vi "Data To API String Arguments.vi"(7 "reference cluster data":variant, 9 "error in (no error)":errorcluster, 10 "No Tag Mode(F)":bool, 11 "data":variant) -> (1 "error out":errorcluster, 3 "String":string)   [LabVIEW 2017, in "API String Arguments Support.lvlib"]
uses:
  API String Arguments Support.lvlib
  <userlib>/_NEVSTOP/Communicable State Machine(CSM)/AdvanceAPI/CSM - Keywords.vi
  <vilib>/Utility/Data Type/NI_Data Type.lvlib
  <userlib>/_NEVSTOP/Communicable State Machine(CSM)/Communicable State Machine.lvlib
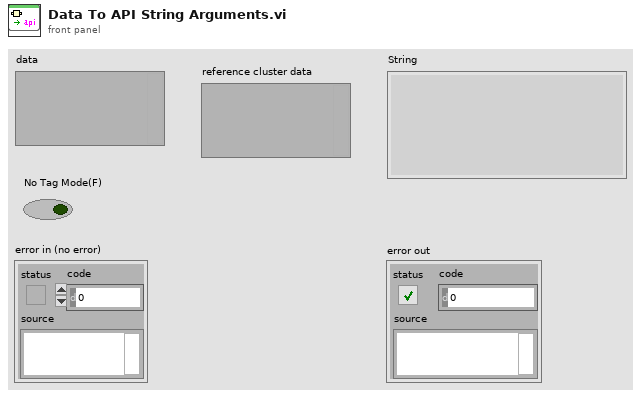
[diagram p1: front panel]
types:
  T1 = typedef "NI_Data Type.lvlib/Data Type.ctl" = enum8{"Invalid Type", "Void", "I8", "I16", "I32", "I64", "U8", "U16", "U32", "U64", "Single Float", "Double Float", "Extended Float", "Single Complex", "Double Complex", "Extended Complex", "Enum U8", "Enum U16", "Enum U32", "Enum U64", "Single Float With Unit", "Double Float With Unit", "Extended Float With Unit", "Single Complex with Unit", "Double Complex with Unit", "Extended Complex with Unit", "Boolean", "String", "Path", "Picture", "Tag", "Array", "Cluster", "Variant", "LV Variant", "Waveform", "Timestamp", "Digital Waveform", "Digital Data", "ExpressData", "Refnum", "External Data", "VI", "Poly VI", "LabVIEW Class Instance", "Fixed Point"}
  T2 = typedef "NI_Data Type.lvlib/Refnum Type.ctl" = enum16{"NotARefnum", "UnknownRefnum", "Generic", "Datalog", "ByteStream", "Device", "Occurence", "TCPNetConnection", "Auto", "Menu", "Imaq", "Hardware", "DataSocket", "Visa", "IVI", "UDPNetConnection", "Notifier", "Queue", "Irda", "EventReg", "DotNet", "UserEvent", "Callback", "UNUSED_EMPTY_POSITION", "BlueToothNetConnection", "LVObjApp", "LVObjVI", "LVObjUnknown", "GenericClass", "UserDefinedRefnumTag", "DataValue", "RT FIFO", "TDMS File"}
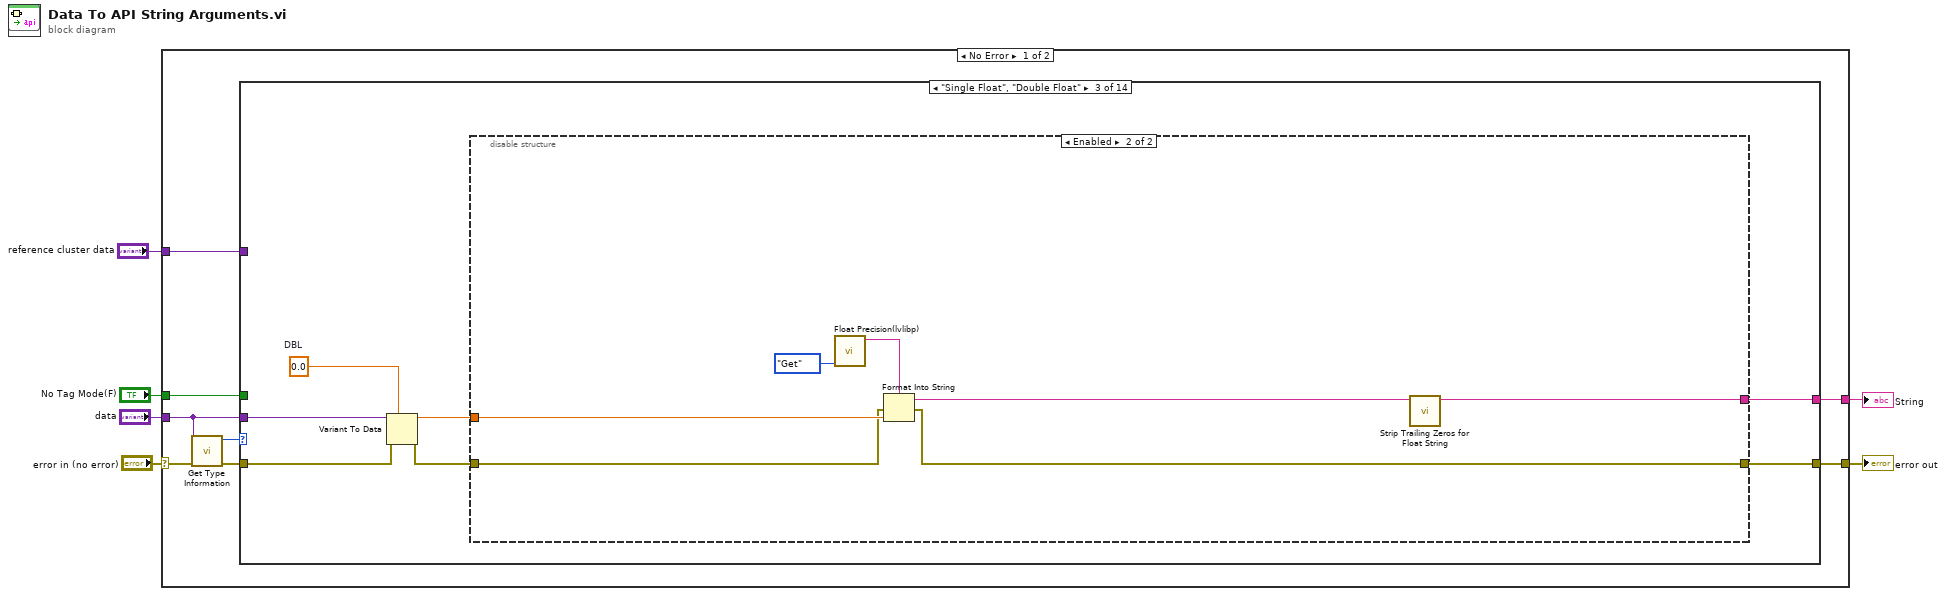
[diagram p0: block diagram]
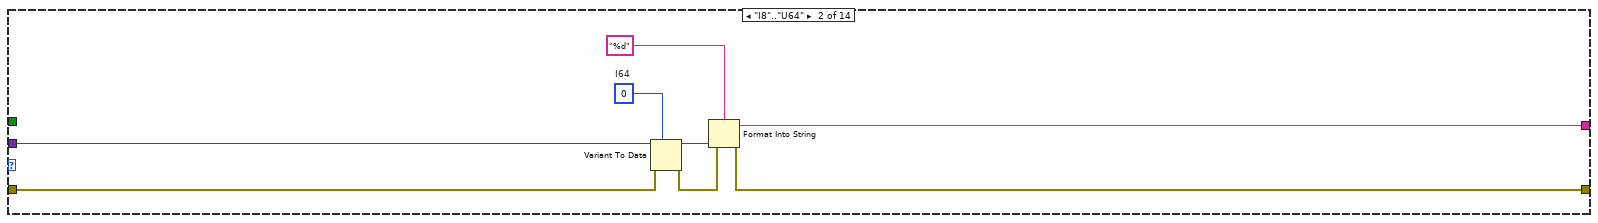
[diagram p3: hidden frame]
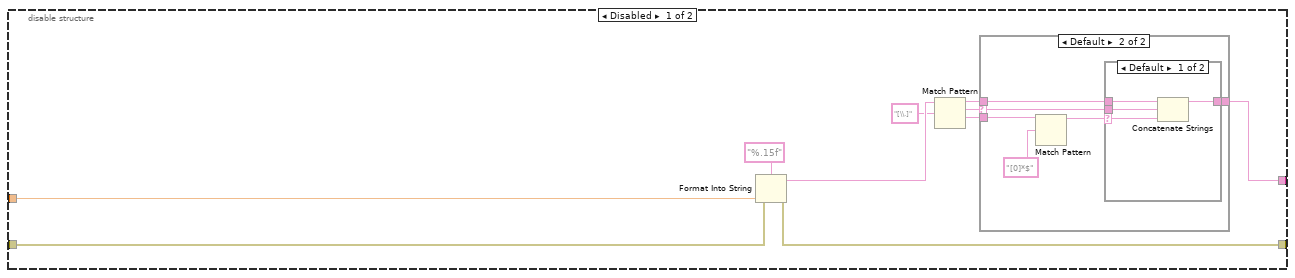
[diagram p4: hidden frame]
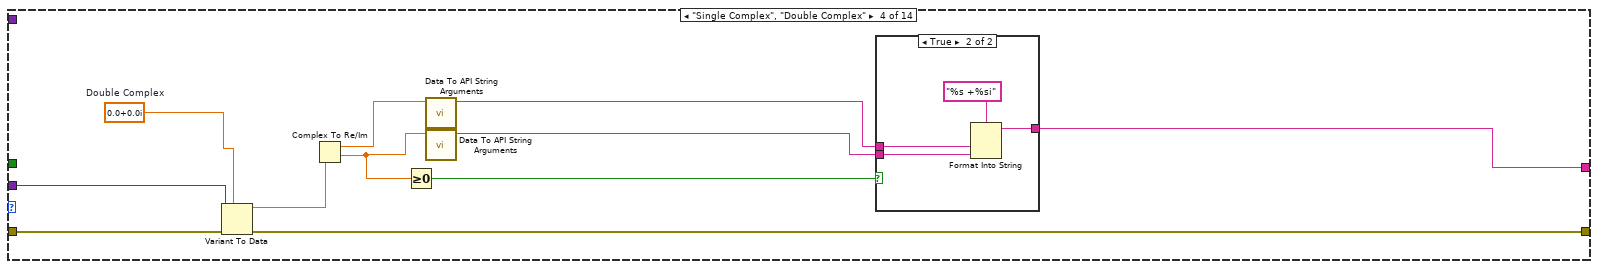
[diagram p7: hidden frame]
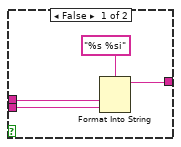
[diagram p8: hidden frame]
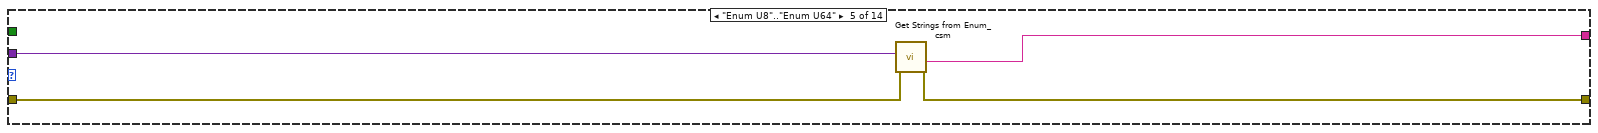
[diagram p9: hidden frame]
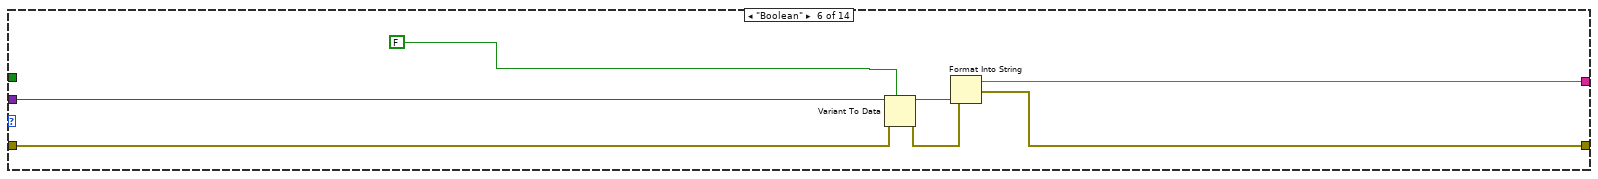
[diagram p10: hidden frame]
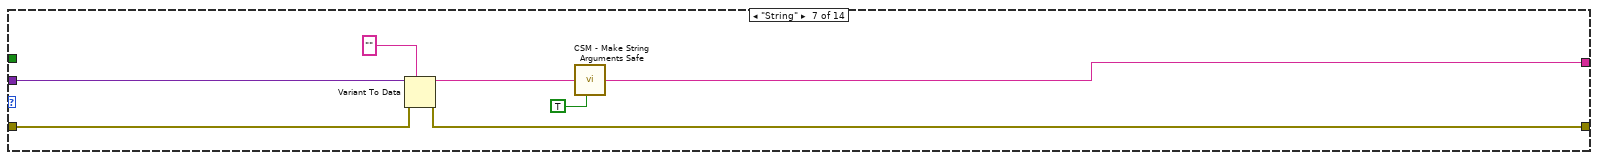
[diagram p11: hidden frame]
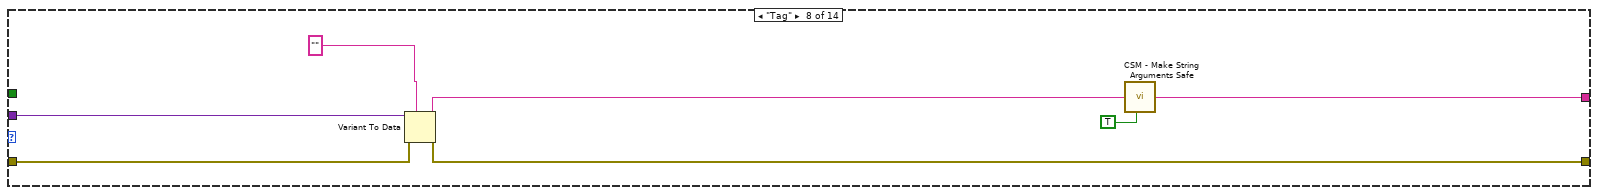
[diagram p12: hidden frame]
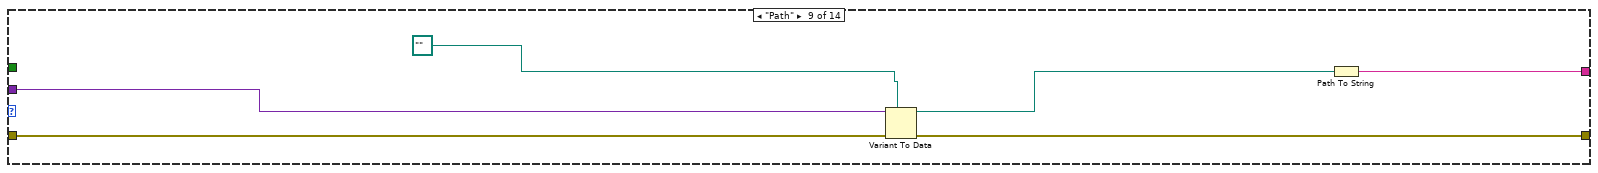
[diagram p13: hidden frame]
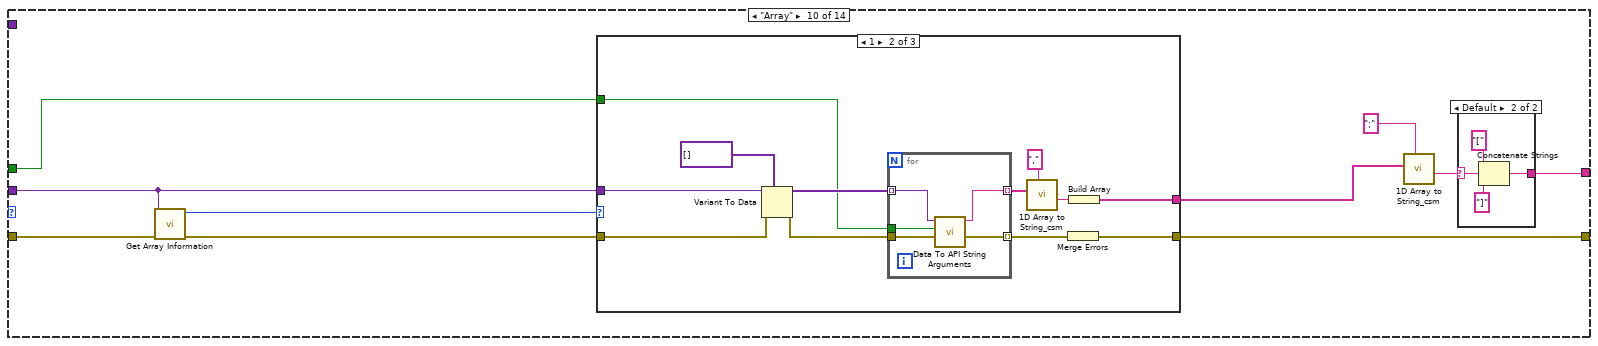
[diagram p14: hidden frame]
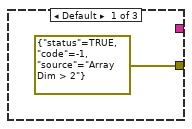
[diagram p15: hidden frame]
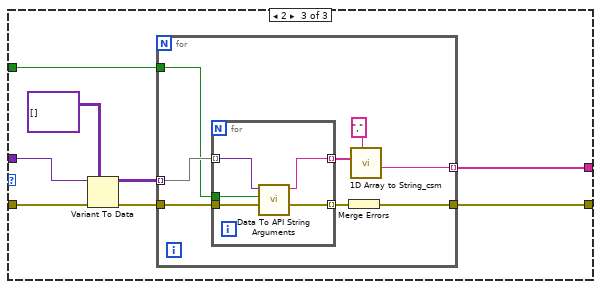
[diagram p16: hidden frame]
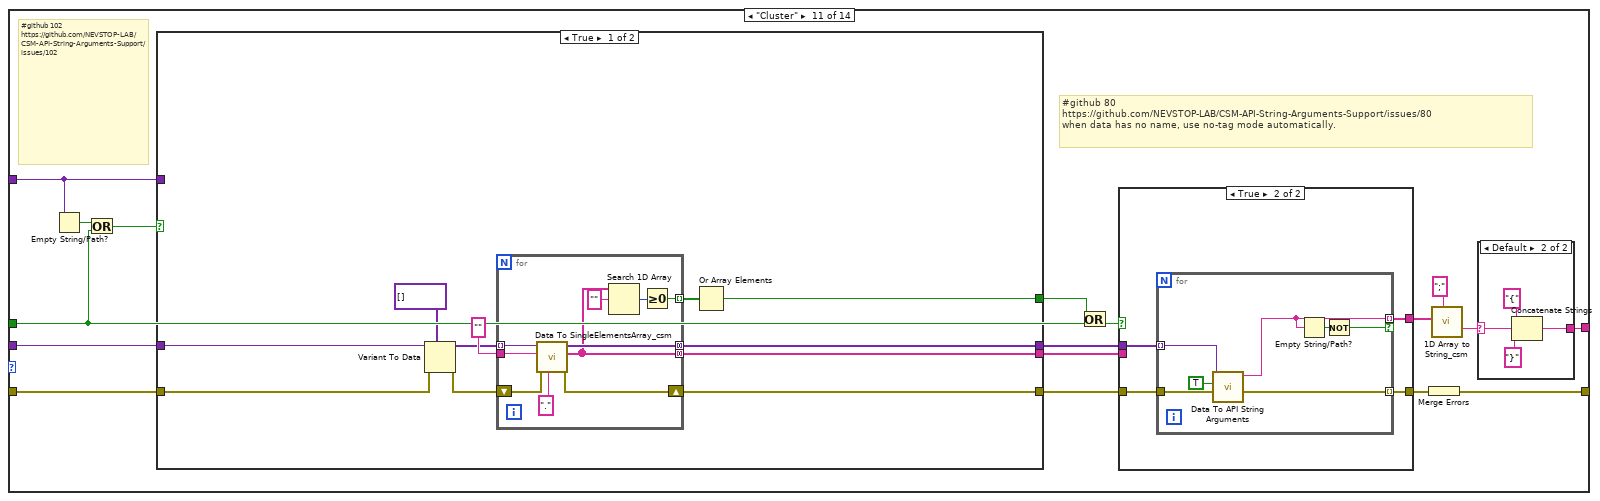
[diagram p18: hidden frame]
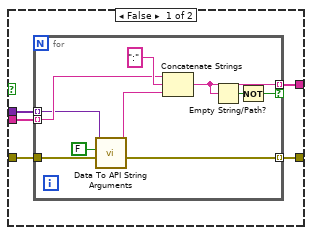
[diagram p19: hidden frame]
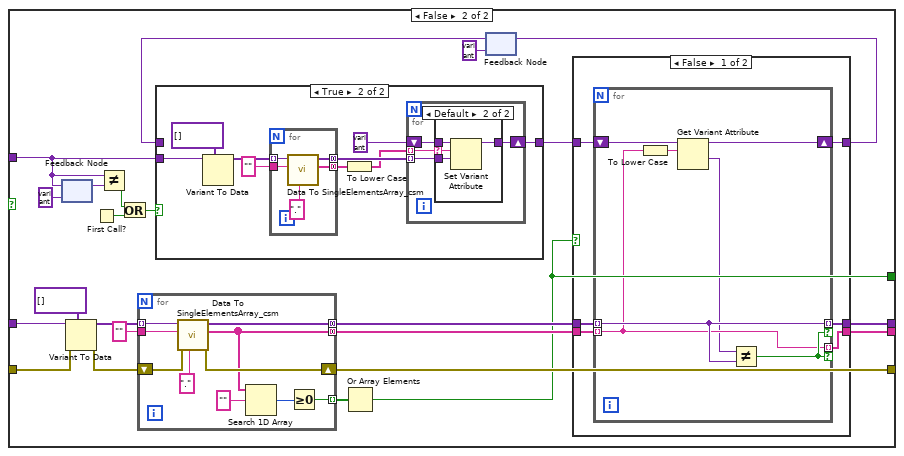
[diagram p20: hidden frame]
diagram:
  n1 = case shown="No Error" "error in (no error)" {
    selector: "error in (no error)" -> [w9 w325]
    tunnel: [w13 _] -> w6
    tunnel: "data" -> [w12 _]
    tunnel: [w10 w325] -> w4
    tunnel: "reference cluster data" -> [w8 _]
    tunnel: "No Tag Mode(F)" -> [w7 _]
    frame No Error {
      n2 = call <vilib>:"Get Type Information.vi"("error in (no error)"=w9, "Variant"=w12) -> ("error out"=w11:errorcluster, "Type"=w14:T1)  [unwired: 5 in, 3 out]
      n3 = case shown="\"Single Float\", \"Double Float\"" w14 {
        tunnel: [_ w19 w24 w65 w81 w87 w91 w98 w104 w119 w179 w304 w310 w319] -> w13
        tunnel: w12 -> [_ w23 w30 w68 w82 w89 w96 w103 w109 w117 w174 w305 w308 w324]
        tunnel: w11 -> [w15 w18 w28 w70 w80 w86 w94 w101 w107 w118 w173 w306 w311 w322]
        tunnel: [w15 w16 w26 w69 w79 w84 w93 w100 w106 w115 w177 w306 w309 w321] -> w10
        tunnel: w8 -> [_ _ _ _ _ _ _ _ _ _ w169 _ _ _]
        tunnel: w7 -> [_ _ _ _ _ _ _ _ _ w110 w163 _ _ _]
        frame "Invalid Type", "Void" {
        }
        frame "I8".."U64" {
          w22 = i64 0  # I64
          n4 = Variant To Data(error in=w18, type=w22, Variant=w23) -> (data=w21:i64, error out=w17:errorcluster)
          n5 = Format Into String(format string="%d", error in=w17, w21) -> (resulting string=w19:string, error out=w16:errorcluster)  [unwired: 1 in]
        }
        frame "Single Float", "Double Float" {
          w25 = 0.0  # DBL
          n6 = Variant To Data(error in=w28, type=w25, Variant=w30) -> (data=w29:dbl, error out=w27:errorcluster)
          n7 = disable-structure shown="Enabled" {
            disable-tunnel: w29 -> [w40 w59]
            disable-tunnel: w27 -> [w38 w58]
            disable-tunnel: [w37 w57] -> w26
            disable-tunnel: [w31 w55] -> w24
            frame Disabled {
              n8 = Format Into String(format string="%.15f", error in=w38, w40) -> (resulting string=w36:string, error out=w37:errorcluster)  [unwired: 1 in]
              n9 = Match Pattern(string=w36, regular expression="[\\.]") -> (before substring=w33:string, match substring=w32:string, after substring=w34:string)  [unwired: 1 in, 1 out]
              n10 = case shown="Default" w32 {
                selector: w32 -> [_ w44]
                tunnel: w34 -> [_ w47]
                tunnel: w33 -> [w41 w45]
                tunnel: [w41 w42] -> w31
                frame "" {
                }
                frame Default {
                  n11 = Match Pattern(string=w47, regular expression="[0]*$") -> (before substring=w43:string)  [unwired: 1 in, 3 out]
                  n12 = case shown="Default" w43 {
                    selector: w43 -> [w49 _]
                    tunnel: w45 -> [w51 w52]
                    tunnel: w44 -> [w50 _]
                    tunnel: [w48 w52] -> w42
                    frame Default {
                      n13 = Concatenate Strings(w51, w50, w49) -> (w48:string)
                    }
                    frame "" {
                    }
                  }
                }
              }
            }
            frame Enabled {
              n14 = call "Float Precision(lvlibp).vi"("Enum"=enum16{"Set", "Get"}."Get") -> ("Format String"=w53:string)  [unwired: 10 in]
              n15 = Format Into String(format string=w53, error in=w58, w59) -> (resulting string=w56:string, error out=w57:errorcluster)  [unwired: 1 in]
              n16 = call "Strip Trailing Zeros for Float String.vi"("Float String"=w56) -> ("Float String with Same Value"=w55:string)  [unwired: 10 in]
            }
          }
        }
        frame "Single Complex", "Double Complex" {
          w67 = cdb 0.0+0.0i  # Double Complex
          n17 = Variant To Data(error in=w70, type=w67, Variant=w68) -> (data=w66:cdb, error out=w69:errorcluster)
          n18 = Complex To Re/Im(x + iy=w66) -> (x=w63:dbl, y=w62:dbl)
          n19 = Greater Or Equal To 0?(x=w62) -> (x >= 0?=w64:bool)
          n20 = call "Data To API String Arguments.vi"("data"=w63) -> ("String"=w61:string)  [unwired: 9 in, 1 out]
          n21 = call "Data To API String Arguments.vi"("data"=w62) -> ("String"=w60:string)  [unwired: 9 in, 1 out]
          n22 = case shown="True" w64 {
            tunnel: w61 -> [w72 w77]
            tunnel: w60 -> [w71 w76]
            tunnel: [w73 w75] -> w65
            frame False {
              n23 = Format Into String(format string="%s %si", w72, w71) -> (resulting string=w73:string)  [unwired: 2 in, 1 out]
            }
            frame True {
              n24 = Format Into String(format string="%s +%si", w77, w76) -> (resulting string=w75:string)  [unwired: 2 in, 1 out]
            }
          }
        }
        frame "Enum U8".."Enum U64" {
          n25 = call <userlib>:"Get Strings from Enum_csm.vi"("error in (no error)"=w80, "Enum"=w82) -> ("error out"=w79:errorcluster, "String Value"=w81:string)  [unwired: 6 in, 2 out]
        }
        frame "Boolean" {
          n26 = Variant To Data(error in=w86, type=FALSE, Variant=w89) -> (data=w88:bool, error out=w85:errorcluster)
          n27 = Format Into String(error in=w85, w88) -> (resulting string=w87:string, error out=w84:errorcluster)  [unwired: 2 in]
        }
        frame "String" {
          n28 = Variant To Data(error in=w94, type="", Variant=w96) -> (data=w95:string, error out=w93:errorcluster)
          n29 = call <userlib>:"CSM - Make String Arguments Safe.vi"("Argument String"=w95, "Ignore Argument Type(F)"=TRUE) -> ("Safe Argument String"=w91:string)  [unwired: 7 in]
        }
        frame "Tag" {
          n30 = Variant To Data(error in=w101, type="", Variant=w103) -> (data=w102:string, error out=w100:errorcluster)
          n31 = call <userlib>:"CSM - Make String Arguments Safe.vi"("Argument String"=w102, "Ignore Argument Type(F)"=TRUE) -> ("Safe Argument String"=w98:string)  [unwired: 7 in]
        }
        frame "Path" {
          n32 = Variant To Data(error in=w107, type=path "", Variant=w109) -> (data=w108:path, error out=w106:errorcluster)
          n33 = Path To String(path=w108) -> (string=w104:string)
        }
        frame "Array" {
          n34 = call <vilib>:"Get Array Information.vi"("error in (no error)"=w118, "Variant"=w117) -> ("error out"=w111:errorcluster, "Number of Dimensions"=w116:i32)  [unwired: 6 in, 2 out]
          n35 = case shown="1" w116 {
            tunnel: [errorcluster {"status"=TRUE, "code"=-1, "source"="Array Dim > 2"} ("error IO") w128 w143] -> w115
            tunnel: [_ w127 w145] -> w113
            tunnel: w117 -> [_ w125 w144]
            tunnel: w111 -> [_ w123 w142]
            tunnel: w110 -> [_ w121 w138]
            frame Default {
            }
            frame 1 {
              n36 = Variant To Data(error in=w123, type=variant[] [], Variant=w125) -> (data=w124:variant[], error out=w122:errorcluster)
              n37 = for {
                tunnel: w124 -> [w137] mode=indexing
                tunnel: w122 -> [w135]
                tunnel: [w136] -> w132 mode=indexing
                tunnel: [w134] -> w131 mode=indexing
                tunnel: w121 -> [w133]
                n38 = call "Data To API String Arguments.vi"("error in (no error)"=w135, "No Tag Mode(F)"=w133, "data"=w137) -> ("error out"=w136:errorcluster, "String"=w134:string)  [unwired: 7 in]
              }
              n39 = call <userlib>:"1D Array to String_csm.vi"("delimiter (Tab)"=",", "Array of Strings"=w131) -> ("delimited string"=w129:string)  [unwired: 9 in]
              n40 = Merge Errors(w132) -> (w128:errorcluster)
              n41 = Build Array(w129) -> (w127:string[])
            }
            frame 2 {
              n42 = Variant To Data(error in=w142, type=variant[][] [], Variant=w144) -> (data=w139:variant[][], error out=w140:errorcluster)
              n43 = for {
                tunnel: [w151] -> w145 mode=indexing
                tunnel: [w150] -> w143
                tunnel: w140 -> [w148]
                tunnel: w139 -> [w147] mode=indexing
                tunnel: w138 -> [w146]
                n44 = for {
                  tunnel: w147 -> [w158] mode=indexing
                  tunnel: w148 -> [w156]
                  tunnel: [w157] -> w149 mode=indexing
                  tunnel: [w155] -> w153 mode=indexing
                  tunnel: w146 -> [w154]
                  n45 = call "Data To API String Arguments.vi"("error in (no error)"=w156, "No Tag Mode(F)"=w154, "data"=w158) -> ("error out"=w157:errorcluster, "String"=w155:string)  [unwired: 7 in]
                }
                n46 = Merge Errors(w149) -> (w150:errorcluster)
                n47 = call <userlib>:"1D Array to String_csm.vi"("delimiter (Tab)"=",", "Array of Strings"=w153) -> ("delimited string"=w151:string)  [unwired: 9 in]
              }
            }
          }
          n48 = call <userlib>:"1D Array to String_csm.vi"("delimiter (Tab)"=";", "Array of Strings"=w113) -> ("delimited string"=w112:string)  [unwired: 9 in]
          n49 = case shown="Default" w112 {
            selector: w112 -> [_ w159]
            tunnel: [_ w162] -> w119
            frame "" {
            }
            frame Default {
              n50 = Concatenate Strings("[" ("string"), w159, "]" ("string")) -> (w162:string)
            }
          }
        }
        frame "Cluster" {
          # "#github 102\nhttps://github.com/NEVSTOP-LAB/CSM-API-String-Arguments-Support/issues/102"
          # "#github 80\nhttps://github.com/NEVSTOP-LAB/CSM-API-String-Arguments-Support/issues/80\nwhen data has no name, use no-tag mode automatically."
          n51 = Empty String/Path?(string/path=w169) -> (empty?=w164:bool)
          n52 = Or(x=w164, y=w163) -> (x .or. y?=w165:bool)
          n53 = case shown="True" w165 {
            tunnel: w174 -> [w212 w245]
            tunnel: w173 -> [w211 w244]
            tunnel: [w210 w242] -> w172
            tunnel: [w209 w239] -> w171
            tunnel: [w208 w240] -> w170
            tunnel: w169 -> [_ w237]
            tunnel: [w206 w230] -> w166
            frame True {
              n54 = Variant To Data(error in=w211, type=variant[] [] ("Array"), Variant=w212) -> (data=w214:variant[], error out=w213:errorcluster)
              n55 = for {
                tunnel: [w224] -> w210 mode=concatenating
                tunnel: [w220] -> w208 mode=concatenating
                tunnel: "" ("parentUrl") -> [w222]
                tunnel: w214 -> [w221] mode=indexing
                shift-right: [w223] -> w209
                shift-left: w213 -> [w226]
                tunnel: [w217] -> w207 mode=indexing
                n56 = call "Data To SingleElementsArray_csm.vi"("Seperator(/)"=".", "error in (no error)"=w226, "parentUrl"=w222, "Cluster"=w221) -> ("error out"=w223:errorcluster, "Full NameList"=w220:string[], "DataElementArray"=w224:variant[])  [unwired: 5 in]
                n57 = Search 1D Array(1D array=w220, element="" ("parentUrl")) -> (index of element=w218:i32)  [unwired: 1 in]
                n58 = Greater Or Equal To 0?(x=w218) -> (x >= 0?=w217:bool)
              }
              n59 = Or Array Elements(Boolean array=w207) -> (logical OR=w206:bool)
            }
            frame False {
              n60 = feedback-in #1(w237) -> ()
              n61 = feedback #1(variant ("reference cluster data")) -> (w236:variant)
              n62 = Variant To Data(error in=w244, type=variant[] [] ("Array"), Variant=w245) -> (data=w247:variant[], error out=w246:errorcluster)
              n63 = First Call?() -> (First Call?: T/F=w235:bool)
              n64 = Not Equal?(x=w237, y=w236) -> (x != y?=w234:bool)
              n65 = Or(x=w234, y=w235) -> (x .or. y?=w233:bool)
              n66 = for {
                tunnel: [w297] -> w243 mode=concatenating
                tunnel: [w291] -> w241 mode=concatenating
                tunnel: "" ("parentUrl") -> [w295]
                tunnel: w247 -> [w294] mode=indexing
                shift-right: [w296] -> w239
                shift-left: w246 -> [w299]
                tunnel: [w290] -> w238 mode=indexing
                n67 = call "Data To SingleElementsArray_csm.vi"("Seperator(/)"=".", "error in (no error)"=w299, "parentUrl"=w295, "Cluster"=w294) -> ("error out"=w296:errorcluster, "Full NameList"=w291:string[], "DataElementArray"=w297:variant[])  [unwired: 5 in]
                n68 = Search 1D Array(1D array=w291, element="" ("parentUrl")) -> (index of element=w293:i32)  [unwired: 1 in]
                n69 = Greater Or Equal To 0?(x=w293) -> (x >= 0?=w290:bool)
              }
              n70 = Or Array Elements(Boolean array=w238) -> (logical OR=w230:bool)
              n71 = feedback #2(variant ("variant")) -> (w232:variant)
              n72 = case shown="True" w233 {
                tunnel: w237 -> [_ w269]
                tunnel: [w266 w268] -> w231
                tunnel: w232 -> [w266 _]
                frame False {
                }
                frame True {
                  n73 = Variant To Data(type=variant[] [] ("Array"), Variant=w269) -> (data=w275:variant[])  [unwired: 1 in, 1 out]
                  n74 = for {
                    tunnel: [w288] -> w272 mode=concatenating
                    tunnel: [w287] -> w271 mode=concatenating
                    tunnel: "" ("parentUrl") -> [w286]
                    tunnel: w275 -> [w285] mode=indexing
                    n75 = call "Data To SingleElementsArray_csm.vi"("Seperator(/)"=".", "parentUrl"=w286, "Cluster"=w285) -> ("Full NameList"=w287:string[], "DataElementArray"=w288:variant[])  [unwired: 6 in, 1 out]
                  }
                  n76 = To Lower Case(string=w271) -> (all lower case string=w267:string[])
                  n77 = for {
                    tunnel: w272 -> [w279] mode=indexing
                    tunnel: w267 -> [w278] mode=indexing
                    shift-right: [w276] -> w268
                    shift-left: variant ("variant") -> [w277]
                    n78 = case shown="Default" w278 {
                      selector: w278 -> [_ w283]
                      tunnel: w279 -> [_ w284]
                      tunnel: w277 -> [w280 w282]
                      tunnel: [w280 w281] -> w276
                      frame "" {
                      }
                      frame Default {
                        n79 = Set Variant Attribute(Variant=w282, name=w283, value=w284) -> (Variant out=w281:variant)  [unwired: 1 in, 2 out]
                      }
                    }
                  }
                }
              }
              n80 = case shown="False" w230 {
                tunnel: w243 -> [w255 w264]
                tunnel: [w254 w264] -> w242
                tunnel: w241 -> [w253 w265]
                tunnel: [w252 w265] -> w240
                tunnel: w231 -> [w251 w263]
                tunnel: [w250 w263] -> w229
                frame False {
                  n81 = for {
                    tunnel: w255 -> [w262] mode=indexing
                    tunnel: w253 -> [w258] mode=indexing
                    tunnel: [w262] -> w254 mode=indexing if=w261
                    tunnel: [w258] -> w252 mode=indexing if=w261
                    shift-right: [w259] -> w250
                    shift-left: w251 -> [w260]
                    n82 = To Lower Case(string=w258) -> (all lower case string=w256:string)
                    n83 = Get Variant Attribute(Variant=w260, name=w256) -> (duplicate Variant=w259:variant, value=w257:variant)  [unwired: 2 in, 2 out]
                    n84 = Not Equal?(x=w257, y=w262) -> (x != y?=w261:bool)
                  }
                }
                frame True {
                }
              }
              n85 = feedback-in #2(w229) -> ()
            }
          }
          n86 = Or(x=w166, y=w163) -> (x .or. y?=w167:bool)
          n87 = case shown="True" w167 {
            tunnel: [w184 w198] -> w178
            tunnel: w172 -> [w183 w197]
            tunnel: w171 -> [w182 w196]
            tunnel: w170 -> [w181 _]
            tunnel: [w180 w195] -> w168
            frame False {
              n88 = for {
                tunnel: [w189] -> w184 mode=indexing
                tunnel: [w188] -> w180 mode=indexing if=w186
                tunnel: w183 -> [w192] mode=indexing
                tunnel: w182 -> [w190]
                tunnel: w181 -> [w193] mode=indexing
                n89 = call "Data To API String Arguments.vi"("error in (no error)"=w190, "No Tag Mode(F)"=FALSE ("No Tag(F)"), "data"=w192) -> ("error out"=w189:errorcluster, "String"=w191:string)  [unwired: 7 in]
                n90 = Concatenate Strings(w193, ":" ("string"), w191) -> (w188:string)
                n91 = Empty String/Path?(string/path=w188) -> (empty?=w187:bool)
                n92 = Not(x=w187) -> (.not. x?=w186:bool)
              }
            }
            frame True {
              n93 = for {
                tunnel: [w203] -> w198 mode=indexing
                tunnel: [w200] -> w195 mode=indexing if=w201
                tunnel: w197 -> [w205] mode=indexing
                tunnel: w196 -> [w204]
                n94 = call "Data To API String Arguments.vi"("error in (no error)"=w204, "No Tag Mode(F)"=TRUE ("No Tag(F)"), "data"=w205) -> ("error out"=w203:errorcluster, "String"=w200:string)  [unwired: 7 in]
                n95 = Empty String/Path?(string/path=w200) -> (empty?=w202:bool)
                n96 = Not(x=w202) -> (.not. x?=w201:bool)
              }
            }
          }
          n97 = Merge Errors(w178) -> (w177:errorcluster)
          n98 = call <userlib>:"1D Array to String_csm.vi"("delimiter (Tab)"=";", "Array of Strings"=w168) -> ("delimited string"=w175:string)  [unwired: 9 in]
          n99 = case shown="Default" w175 {
            selector: w175 -> [_ w300]
            tunnel: [_ w303] -> w179
            frame "" {
            }
            frame Default {
              n100 = Concatenate Strings("{" ("string"), w300, "}" ("string")) -> (w303:string)
            }
          }
        }
        frame Default {
          n101 = call <userlib>:"CSM - Convert Data to HexStr.vi"("Variant"=w305) -> ("HEX String (0-9,A-F)"=w304:string)  [unwired: 8 in]
        }
        frame "Refnum" {
          n102 = call <vilib>:"Get Refnum Information.vi"("error in (no error)"=w311, "Variant"=w308) -> ("error out"=w309:errorcluster, "Reference Type"=w307:T2)  [unwired: 6 in, 2 out]
          n103 = case shown="\"Visa\", \"IVI\", \"UserDefinedRefnumTag\"" w307 {
            tunnel: [w313 w318] -> w310
            tunnel: w308 -> [w316 w317]
            frame "Visa", "IVI", "UserDefinedRefnumTag" {
              # "UserDefinedRefnumTag\nlike Camera Refnum"
              n104 = Variant To Data(type="" ("HEX String (0-9,A-F)"), Variant=w316) -> (data=w314:string)  [unwired: 1 in, 1 out]
              n105 = call <userlib>:"CSM - Make String Arguments Safe.vi"("Argument String"=w314, "Ignore Argument Type(F)"=TRUE) -> ("Safe Argument String"=w313:string)  [unwired: 7 in]
            }
            frame Default {
              n106 = call <userlib>:"CSM - Convert Data to HexStr.vi"("Variant"=w317) -> ("HEX String (0-9,A-F)"=w318:string)  [unwired: 8 in]
            }
          }
        }
        frame "Timestamp" {
          n107 = Variant To Data(error in=w322, type=timestamp(0 s since 1904-01-01) ("Timestamp (now)"), Variant=w324) -> (data=w320:timestamp, error out=w321:errorcluster)
          n108 = call "CSM - Timestamp to API String Arguments.vi"("Timestamp (now)"=w320) -> ("API String"=w319:string)  [unwired: 9 in, 1 out]
        }
      }
    }
    frame Error {
    }
  }
  "String" <- w6
  "error out" <- w4
